vi "Tabellen Index Manager.vi"(0 "Spangaseinstellungen":T1[](array[typedef]) {"Komponenten"."Komponente 5"."Komponente:" items=["NO (350,3000) LP 191C", "NO2 (150) LP 191C (1of2)", "NO2 (2000) LP 191C (2of2)", "N2O (300) LP 191C (1of2)", "NH3 (300) LP 191C (1of2)", "NH3 (900,3000) LP 191C (2of2)", "HNCO (400) 191C", "H2O% (30) LP 191C", "Formaldehyde (70,500) LP 191C", "CO2 low% (4) LP 191C (2of2)", "CO2% (20) LP 191C (1of2)", "CO (700) LP 191C (1of3)", "CO% (1) LP 191C (2of3)", "Propylene (1000) LP 191C", "Aromatic HC C7 (500) LP 191C", "Ethylene (1000) LP 191C", "CH4 (250) LP 191C (1of2)", "CH4 (5000) LP 191C (2of2)", "Ethane (1000) LP 191C", "Acetylene (1000) LP 191C", "HNO2 (20) 191C", "MeOH (1000) 191C", "CO% (10) LP 191C (3of3)", "Formic Acid (100) 191C", "SO2 (500) LP 191C", "Acetaldehyde (1000) LP 191C", "COS (100) LP 191C", "1,3 butadiene (100) LP 191C", "Oil as Octane (200) LP 191C", "N2O (1000) LP 191C (2of2)", "Propane (200) LP 191C", "NO2 autorange (2000)", "CO autorange (100000)", "CH4 autorange (5000)", "NH3 autorange (3000)", "Temp. Gascell", "Pressure Gascell", "sBeam@2500"]; "Komponenten"."Komponente 5"."Konzentration IST" format="%#.4f"; "Komponenten"."Komponente 5"."Genauigkeit" format="%#.1f"; "Komponenten"."Komponente 4"."Komponente:" items=["NO (350,3000) LP 191C", "NO2 (150) LP 191C (1of2)", "NO2 (2000) LP 191C (2of2)", "N2O (300) LP 191C (1of2)", "NH3 (300) LP 191C (1of2)", "NH3 (900,3000) LP 191C (2of2)", "HNCO (400) 191C", "H2O% (30) LP 191C", "Formaldehyde (70,500) LP 191C", "CO2 low% (4) LP 191C (2of2)", "CO2% (20) LP 191C (1of2)", "CO (700) LP 191C (1of3)", "CO% (1) LP 191C (2of3)", "Propylene (1000) LP 191C", "Aromatic HC C7 (500) LP 191C", "Ethylene (1000) LP 191C", "CH4 (250) LP 191C (1of2)", "CH4 (5000) LP 191C (2of2)", "Ethane (1000) LP 191C", "Acetylene (1000) LP 191C", "HNO2 (20) 191C", "MeOH (1000) 191C", "CO% (10) LP 191C (3of3)", "Formic Acid (100) 191C", "SO2 (500) LP 191C", "Acetaldehyde (1000) LP 191C", "COS (100) LP 191C", "1,3 butadiene (100) LP 191C", "Oil as Octane (200) LP 191C", "N2O (1000) LP 191C (2of2)", "Propane (200) LP 191C", "NO2 autorange (2000)", "CO autorange (100000)", "CH4 autorange (5000)", "NH3 autorange (3000)", "Temp. Gascell", "Pressure Gascell", "sBeam@2500"]; "Komponenten"."Komponente 4"."Konzentration IST" format="%#.4f"; "Komponenten"."Komponente 4"."Genauigkeit" format="%#.1f"; "Komponenten"."Komponente 3"."Komponente:" items=["NO (350,3000) LP 191C", "NO2 (150) LP 191C (1of2)", "NO2 (2000) LP 191C (2of2)", "N2O (300) LP 191C (1of2)", "NH3 (300) LP 191C (1of2)", "NH3 (900,3000) LP 191C (2of2)", "HNCO (400) 191C", "H2O% (30) LP 191C", "Formaldehyde (70,500) LP 191C", "CO2 low% (4) LP 191C (2of2)", "CO2% (20) LP 191C (1of2)", "CO (700) LP 191C (1of3)", "CO% (1) LP 191C (2of3)", "Propylene (1000) LP 191C", "Aromatic HC C7 (500) LP 191C", "Ethylene (1000) LP 191C", "CH4 (250) LP 191C (1of2)", "CH4 (5000) LP 191C (2of2)", "Ethane (1000) LP 191C", "Acetylene (1000) LP 191C", "HNO2 (20) 191C", "MeOH (1000) 191C", "CO% (10) LP 191C (3of3)", "Formic Acid (100) 191C", "SO2 (500) LP 191C", "Acetaldehyde (1000) LP 191C", "COS (100) LP 191C", "1,3 butadiene (100) LP 191C", "Oil as Octane (200) LP 191C", "N2O (1000) LP 191C (2of2)", "Propane (200) LP 191C", "NO2 autorange (2000)", "CO autorange (100000)", "CH4 autorange (5000)", "NH3 autorange (3000)", "Temp. Gascell", "Pressure Gascell", "sBeam@2500"]; "Komponenten"."Komponente 3"."Konzentration IST" format="%#.4f"; "Komponenten"."Komponente 3"."Genauigkeit" format="%#.1f"; "Komponenten"."Komponente 2"."Komponente:" items=["NO (350,3000) LP 191C", "NO2 (150) LP 191C (1of2)", "NO2 (2000) LP 191C (2of2)", "N2O (300) LP 191C (1of2)", "NH3 (300) LP 191C (1of2)", "NH3 (900,3000) LP 191C (2of2)", "HNCO (400) 191C", "H2O% (30) LP 191C", "Formaldehyde (70,500) LP 191C", "CO2 low% (4) LP 191C (2of2)", "CO2% (20) LP 191C (1of2)", "CO (700) LP 191C (1of3)", "CO% (1) LP 191C (2of3)", "Propylene (1000) LP 191C", "Aromatic HC C7 (500) LP 191C", "Ethylene (1000) LP 191C", "CH4 (250) LP 191C (1of2)", "CH4 (5000) LP 191C (2of2)", "Ethane (1000) LP 191C", "Acetylene (1000) LP 191C", "HNO2 (20) 191C", "MeOH (1000) 191C", "CO% (10) LP 191C (3of3)", "Formic Acid (100) 191C", "SO2 (500) LP 191C", "Acetaldehyde (1000) LP 191C", "COS (100) LP 191C", "1,3 butadiene (100) LP 191C", "Oil as Octane (200) LP 191C", "N2O (1000) LP 191C (2of2)", "Propane (200) LP 191C", "NO2 autorange (2000)", "CO autorange (100000)", "CH4 autorange (5000)", "NH3 autorange (3000)", "Temp. Gascell", "Pressure Gascell", "sBeam@2500"]; "Komponenten"."Komponente 2"."Konzentration IST" format="%#.4f"; "Komponenten"."Komponente 2"."Genauigkeit" format="%#.1f"; "Komponenten"."Komponente 1"."Komponente:" items=["NO (350,3000) LP 191C", "NO2 (150) LP 191C (1of2)", "NO2 (2000) LP 191C (2of2)", "N2O (300) LP 191C (1of2)", "NH3 (300) LP 191C (1of2)", "NH3 (900,3000) LP 191C (2of2)", "HNCO (400) 191C", "H2O% (30) LP 191C", "Formaldehyde (70,500) LP 191C", "CO2 low% (4) LP 191C (2of2)", "CO2% (20) LP 191C (1of2)", "CO (700) LP 191C (1of3)", "CO% (1) LP 191C (2of3)", "Propylene (1000) LP 191C", "Aromatic HC C7 (500) LP 191C", "Ethylene (1000) LP 191C", "CH4 (250) LP 191C (1of2)", "CH4 (5000) LP 191C (2of2)", "Ethane (1000) LP 191C", "Acetylene (1000) LP 191C", "HNO2 (20) 191C", "MeOH (1000) 191C", "CO% (10) LP 191C (3of3)", "Formic Acid (100) 191C", "SO2 (500) LP 191C", "Acetaldehyde (1000) LP 191C", "COS (100) LP 191C", "1,3 butadiene (100) LP 191C", "Oil as Octane (200) LP 191C", "N2O (1000) LP 191C (2of2)", "Propane (200) LP 191C", "NO2 autorange (2000)", "CO autorange (100000)", "CH4 autorange (5000)", "NH3 autorange (3000)", "Temp. Gascell", "Pressure Gascell", "sBeam@2500"]; "Komponenten"."Komponente 1"."Konzentration IST" format="%#.4f"; "Komponenten"."Komponente 1"."Genauigkeit" format="%#.1f"; "Modus" items=["Cal Gas to PNS", "Cal Gas to Samplepoint"]; "Ablaufdatum" format="%<%d.%m.%Y>T"; "Gasflasche" items=["----"=10000, "IAG NH3 3000"=0, "IAG NH3 200"=1, "IAG NH3 2000"=2, "IAG MG"=3, "IAG O2"=4]}, 11 "error in (no error)":errorcluster caption="Fehler (Eingang, kein Fehler)") -> (4 "Tabellenbeginn":i32[](array[numeric]), 8 "Verwendete Spangaseingänge":i32[](array[numeric]), 15 "error out":errorcluster caption="Fehler (Ausgang)")   [LabVIEW 2020, in "EPA 1065.lvlib" / "Gas Analyzer Drift 1065-550.lvlib"]
uses:
  Gas Analyzer Drift 1065-550.lvlib
  Spaninlet Cluster.ctl
  Seiten/System Einstellungen V2/Konfig Gasflasche.ctl
  Seiten/System Einstellungen V2/Analysatoren.ctl
  Seiten/System Einstellungen V2/Gasflasche Auswahl.ctl
  T90 1065-308/Modus.ctl
  Komponentencluster.ctl
  Komponentenauswahl.ctl
  Seiten/System Einstellungen V2/System Einstellungen V2.lvlib
  T90 1065-308/T90 Test 1065-308.lvlib
panel:
  out "Größen Gasauswahl":i32[](array[numeric])
  # "Komponente"
  # "Konzentration"
  # "Einheit"
  # "Genauigkeit [%]"
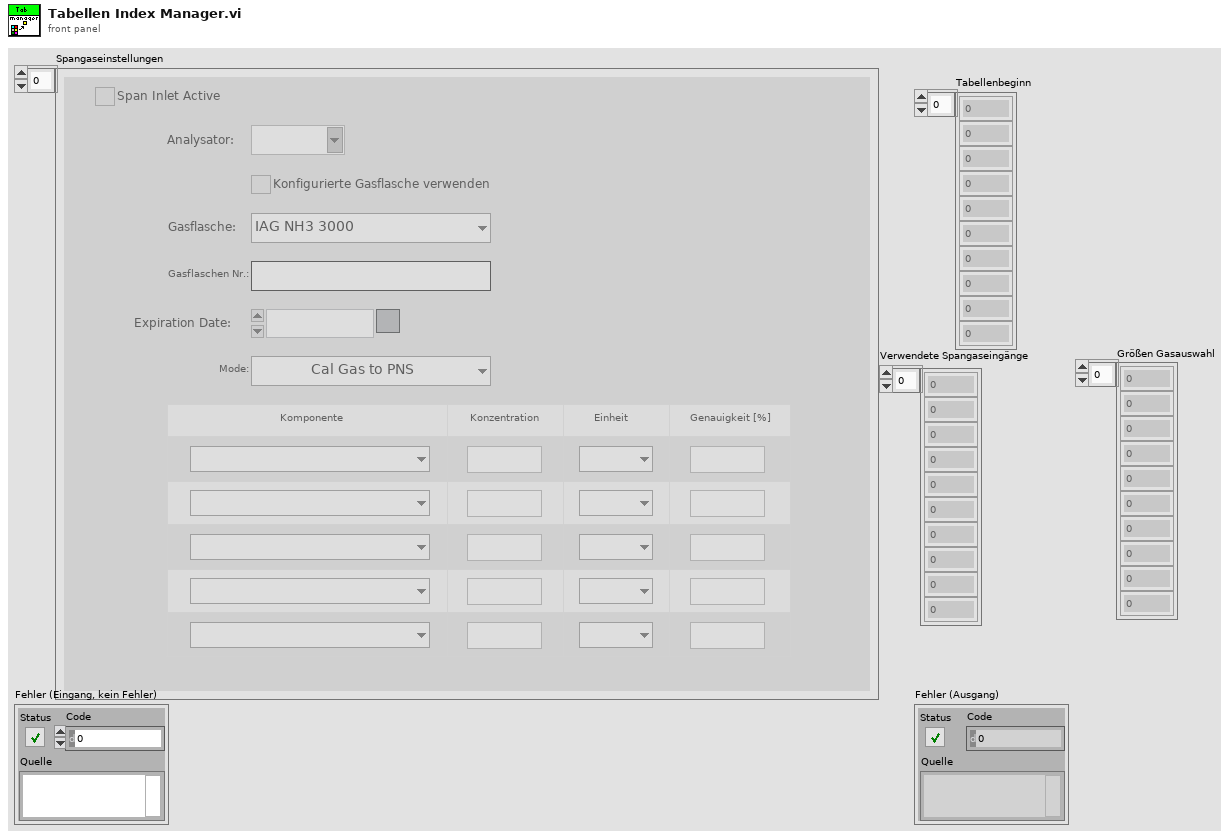
[diagram p1: front panel]
types:
  T1 = typedef "EPA 1065.lvlib/Gas Analyzer Drift 1065-550.lvlib/Spaninlet Cluster.ctl" = cluster{"Span Inlet Active":T2, "Analysator":T3, "Konfig Gasflasche":T2, "Gasflasche":T4, "Gasflaschen Nr.:":string, "Ablaufdatum":timestamp, "Modus":T5, "Komponenten":T6}
  T2 = typedef "System Einstellungen V2.lvlib/Konfig Gasflasche.ctl" = bool
  T3 = typedef "System Einstellungen V2.lvlib/Analysatoren.ctl" = string
  T4 = typedef "System Einstellungen V2.lvlib/Gasflasche Auswahl.ctl" = u16
  T5 = typedef "EPA 1065.lvlib/T90 Test 1065-308.lvlib/Modus.ctl" = u16
  T6 = typedef "EPA 1065.lvlib/Gas Analyzer Drift 1065-550.lvlib/Komponentencluster.ctl" = cluster{"Komponente 1":T7, "Komponente 2":T7, "Komponente 3":T7, "Komponente 4":T7, "Komponente 5":T7}
  T7 = typedef "EPA 1065.lvlib/Gas Analyzer Drift 1065-550.lvlib/Komponentenauswahl.ctl" = cluster{"Komponente:":u16, "Konzentration IST":dbl, "Einheit":enum16{"ppm", "%"}, "Genauigkeit":dbl}
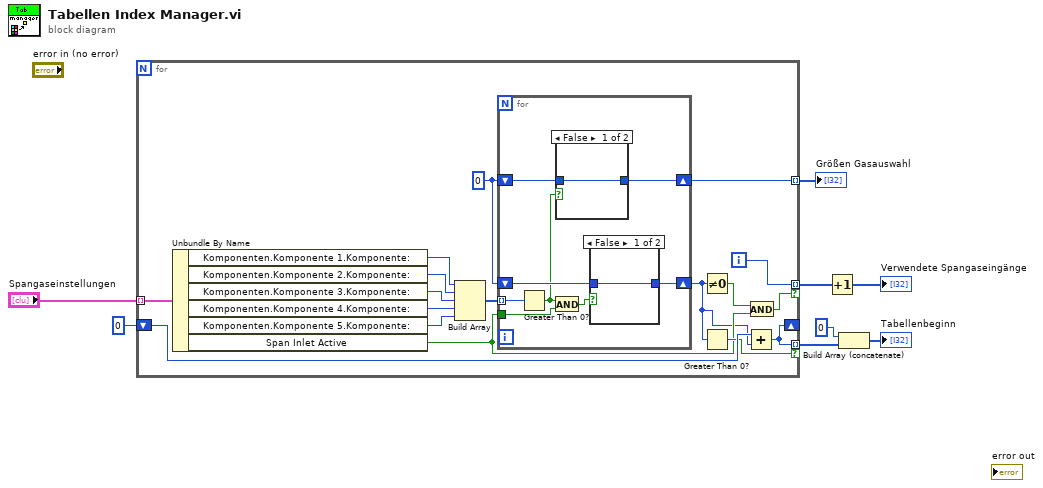
[diagram p0: block diagram]
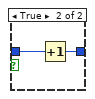
[diagram p2: hidden frame]
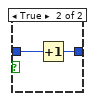
[diagram p3: hidden frame]
diagram:
  n1 = for {
    tunnel: "Spangaseinstellungen" -> [w25] mode=indexing
    shift-right: [w17] -> _
    shift-left: 0 -> [w18]
    tunnel: [w17] -> w1 mode=indexing if=w13
    tunnel: [w16] -> w6 mode=indexing if=w14
    tunnel: [w10] -> w4 mode=indexing
    i -> [w16]
    w11 = 0
    n2 = Unbundle By Name(w25) -> ("Komponenten.Komponente 1.Komponente:"=w24:u16, "Komponenten.Komponente 2.Komponente:"=w23:u16, "Komponenten.Komponente 3.Komponente:"=w22:u16, "Komponenten.Komponente 4.Komponente:"=w21:u16, "Komponenten.Komponente 5.Komponente:"=w20:u16, "Span Inlet Active"=w12:T2)
    n3 = Build Array(w24, w23, w22, w21, w20) -> (w19:u16[])
    n4 = for {
      tunnel: w19 -> [w33] mode=indexing
      shift-right: [w31] -> w9
      shift-left: w11 -> [w32]
      tunnel: w12 -> [w29]
      shift-right: [w27] -> w10
      shift-left: w11 -> [w28]
      n5 = Greater Than 0?(x=w33) -> (x > 0?=w26:bool)
      n6 = And(x=w26, y=w29) -> (x .and. y?=w30:T2)
      n7 = case shown="False" w26 {
        tunnel: w28 -> [w34 w36]
        tunnel: [w34 w35] -> w27
        frame False {
        }
        frame True {
          n8 = Increment(x=w36) -> (x+1=w35:i32)
        }
      }
      n9 = case shown="False" w30 {
        tunnel: w32 -> [w37 w39]
        tunnel: [w37 w38] -> w31
        frame False {
        }
        frame True {
          n10 = Increment(x=w39) -> (x+1=w38:i32)
        }
      }
    }
    n11 = Not Equal To 0?(x=w9) -> (x != 0?=w15:bool)
    n12 = Greater Than 0?(x=w9) -> (x > 0?=w13:bool)
    n13 = Add(x=w18, y=w9) -> (x+y=w17:i32)
    n14 = And(x=w15, y=w12) -> (x .and. y?=w14:T2)
  }
  "Größen Gasauswahl" <- w4
  n15 = Increment(x=w6) -> (x+1=→"Verwendete Spangaseingänge":i32[])
  n16 = Build Array (concatenate)(0, w1) -> (→"Tabellenbeginn":i32[])
